vi "Controller.vi"   [LabVIEW 2013]
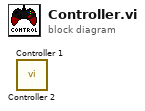
[diagram p0: block diagram]
diagram:
  n1 = call "Controller 2.vi"() -> ()  [unwired: 1 in, 1 out]
  n2 = call "Controller 1.vi"() -> ()  [unwired: 1 in, 1 out]
